vi "z_opti.vi"(6 "error in (no error)":errorcluster, 8 "cam":refnum<queue>, 9 "data":refnum<queue>, 10 "Axis":string(combo), 11 "IP address":string="172.24.192.135") -> (1 "center":dbl, 2 "Y":dbl[](array[numeric]), 3 "X":dbl[](array[numeric]), 4 "error out":errorcluster)   [LabVIEW 2012]
uses:
  <vilib>/Analysis/1siggen.llb/Ramp Pattern by Samples.vi
  <vilib>/Analysis/NI_AALBase.lvlib
  <vilib>/Analysis/NI_AALPro.lvlib
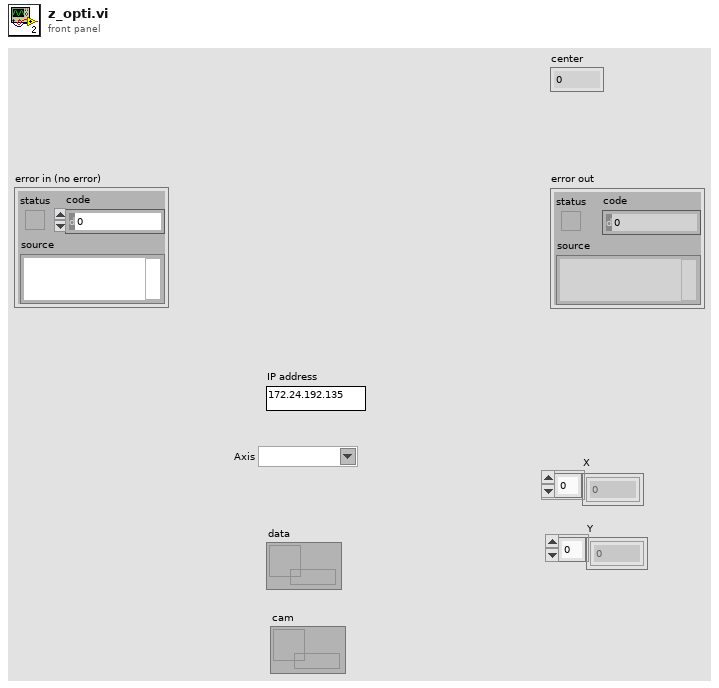
[diagram p1: front panel]
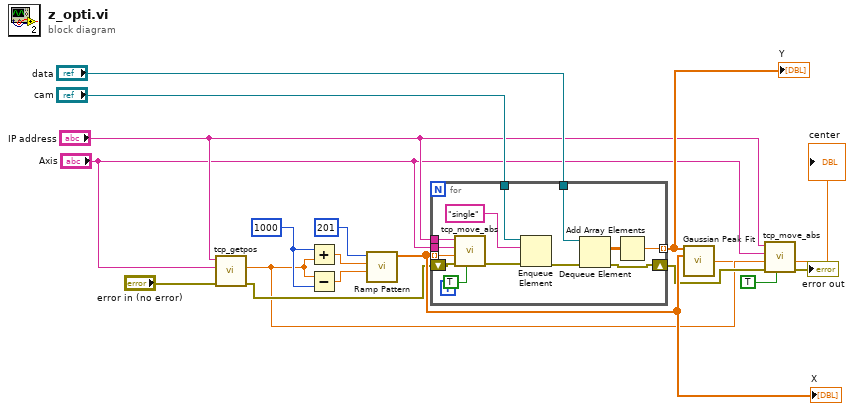
[diagram p0: block diagram]
diagram:
  w16 = 1000
  n1 = call "tcp_getpos.vi"("error in (no error)"="error in (no error)", "Axis"="Axis", "IP address"="IP address") -> ("error out"=w7:errorcluster, "position"=w4:dbl)  [unwired: 6 in, 1 out]
  n2 = Add(x=w16, y=w4) -> (x+y=w2:dbl)
  n3 = Subtract(x=w4, y=w16) -> (x-y=w1:dbl)
  n4 = call-poly <vilib>:"Ramp Pattern.vi"("start"=w1, "end"=w2, "samples"=201) -> ("Ramp Pattern"=w12:dbl[])  [unwired: 7 in, 1 out]
  "X" <- w12
  n5 = for {
    tunnel: w12 -> [w30] mode=indexing
    tunnel: "Axis" -> [w29]
    tunnel: "IP address" -> [w28]
    tunnel: "cam" -> [w24]
    tunnel: "data" -> [w25]
    tunnel: [w20] -> w13 mode=indexing
    shift-right: [w18] -> w6
    shift-left: w7 -> [w19]
    n6 = call "tcp_move_abs.vi"("wait4motiondone"=TRUE, "error in (no error)"=w19, "destination nm/u°"=w30, "Axis"=w29, "IP address"=w28) -> ("error out"=w27:errorcluster)  [unwired: 4 in, 2 out]
    n7 = Enqueue Element(queue=w24, element="single", error in (no error)=w27) -> (error out=w26:errorcluster)  [unwired: 1 in, 2 out]
    n8 = Dequeue Element(queue=w25, error in (no error)=w26) -> (element=w21:dbl[][], error out=w18:errorcluster)  [unwired: 1 in, 2 out]
    n9 = Add Array Elements(numeric array=w21) -> (sum=w20:dbl)
  }
  "Y" <- w13
  n10 = call <vilib>:"Gaussian Peak Fit.vi"("Y"=w13, "X"=w12) -> ("center"=→"center":dbl)  [unwired: 7 in, 6 out]
  n11 = call "tcp_move_abs.vi"("wait4motiondone"=TRUE, "error in (no error)"=w6, "destination nm/u°"=w4, "Axis"="Axis", "IP address"="IP address") -> ("error out"=→"error out":errorcluster)  [unwired: 4 in, 2 out]
